vi "sm i16 write and increment.vi"(9 "Identifier":string, 10 "value in":i16, 11 "Shared memory cluster input":T1) -> (3 "Shared memory cluster output":T1)   [LabVIEW 2020, in "linuxSharedMemory.lvlib"]
uses:
  linuxSharedMemory.lvlib
  controls/sm_cluster.ctl
  <vilib>/NI/NI Linux RT IPC/Shared Memory/Pointer Operations/Write Scalar I16.vi
  <vilib>/NI/NI Linux RT IPC/Shared Memory/Linux RT IPC.Shared Memory.lvlib
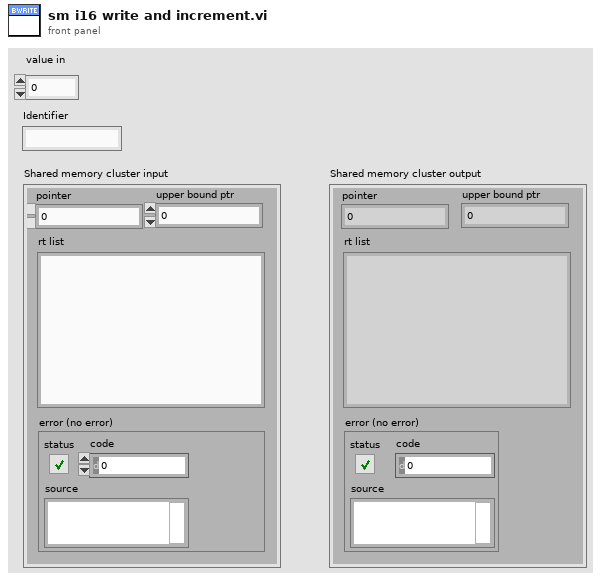
[diagram p1: front panel]
types:
  T1 = typedef "linuxSharedMemory.lvlib/sm_cluster.ctl" = cluster{"rt list":string, "error (no error)":errorcluster, "pointer":u64, "upper bound ptr":u64}
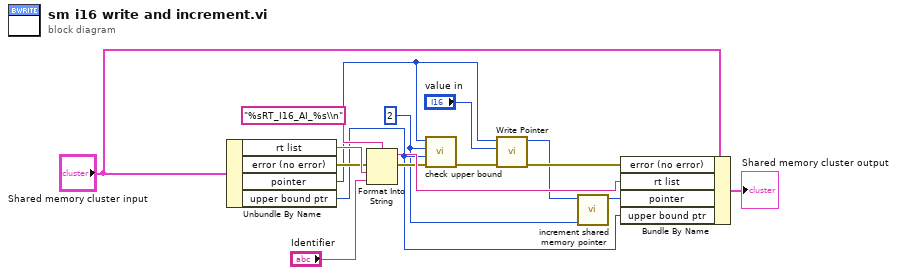
[diagram p0: block diagram]
diagram:
  w1 = 2
  n1 = Unbundle By Name("Shared memory cluster input") -> ("rt list"=w11:string, "error (no error)"=w9:errorcluster, "pointer"=w3:u64, "upper bound ptr"=w6:u64)
  n2 = Format Into String(format string="%sRT_I16_AI_%s\\n", error in=w9, w11, "Identifier") -> (resulting string=w10:string, error out=w8:errorcluster)  [unwired: 1 in]
  n3 = call "check upper bound.vi"("error in (no error)"=w8, "ptr upper bound (inclusive)"=w6, "size"=w1, "ptr in"=w3) -> ("error out"=w5:errorcluster)  [unwired: 7 in]
  n4 = call-poly <vilib>:"Write Pointer.vi"("error in (no error)"=w5, "value"="value in", "pointer in"=w3) -> ("error out"=w4:errorcluster, "pointer out"=w2:u64)  [unwired: 6 in, 1 out]
  n5 = call "increment shared memory pointer.vi"("Increment value"=w1, "Shared Memory PTR in"=w2) -> ("Shared Memory PTR out"=w7:u64)  [unwired: 9 in]
  n6 = Bundle By Name(cluster="Shared memory cluster input", "error (no error)"=w4, "rt list"=w10, "pointer"=w7, "upper bound ptr"=w6) -> (→"Shared memory cluster output":T1)
